vi "XYGo_example.vi"() -> ()   [LabVIEW 2016]
uses:
  Classes/Controller/Motion/A3200 Folder/A3200.lvclass
panel:
  out "Final Position":dbl[](array[numeric])
  out "Initial position":dbl[](array[numeric])
  in  "Speed (mm/s)":dbl=40.0
  in  "XY":dbl[](array[numeric])=[200.0, 300.0]
  # "Input parameter"
  # "Output Current Position"
  # "X\nY"
  # "X\nY\nZ\nU"
  # "1. This example shows how to move gantry to an absolute position on the XY plane with speed specified. \n2. The program would also show the position before and after the moving"
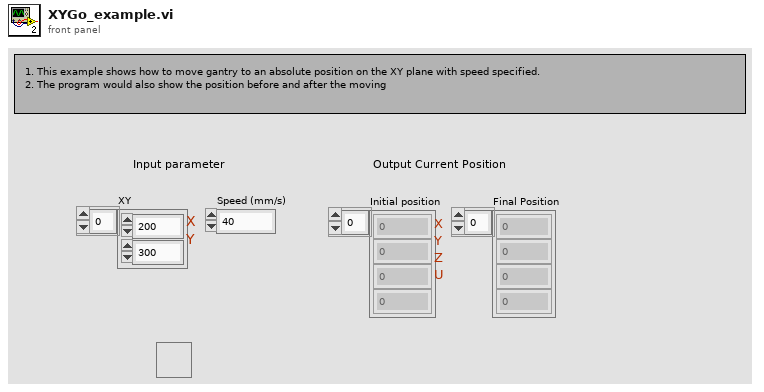
[diagram p1: front panel]
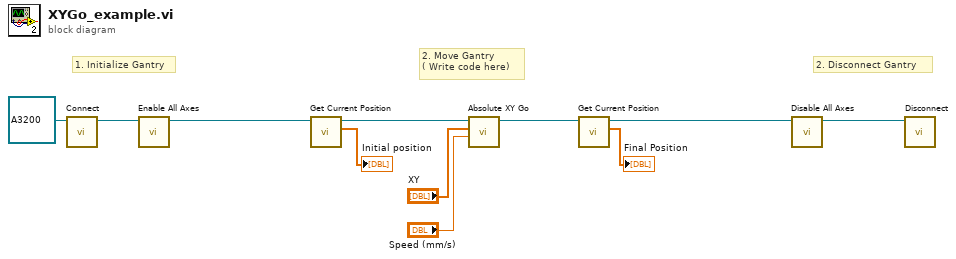
[diagram p0: block diagram]
diagram:
  # "2. Disconnect Gantry"
  # "2. Move Gantry \n( Write code here)"
  # "1. Initialize Gantry"
  n1 = call-dynamic "Connect.vi"("Gantry in"=refnum<class "A3200.lvclass"> refnum ("A3200.lvclass")) -> ("Gantry out"=w10:refnum<class "A3200.lvclass">)  [unwired: 9 in, 1 out]
  n2 = call-dynamic "Enable All Axes.vi"("A3200 in"=w10) -> ("A3200 out"=w6:refnum<class "A3200.lvclass">)  [unwired: 9 in, 1 out]
  n3 = call-dynamic "Get Current Position.vi"("Gantry in"=w6) -> ("XYZTheta Out"=→"Initial position":dbl[], "Gantry out"=w5:refnum<class "A3200.lvclass">)  [unwired: 8 in, 1 out]
  n4 = call-dynamic "Absolute XY Go.vi"("Speed"="Speed (mm/s)", "XY"="XY", "Gantry in"=w5) -> ("Gantry out"=w3:refnum<class "A3200.lvclass">)  [unwired: 7 in, 1 out]
  n5 = call-dynamic "Get Current Position.vi"("Gantry in"=w3) -> ("XYZTheta Out"=→"Final Position":dbl[], "Gantry out"=w2:refnum<class "A3200.lvclass">)  [unwired: 8 in, 1 out]
  n6 = call-dynamic "Disable All Axes.vi"("Gantry in"=w2) -> ("Gantry out"=w9:refnum<class "A3200.lvclass">)  [unwired: 9 in, 1 out]
  n7 = call-dynamic "Disconnect.vi"("Gantry in"=w9) -> ()  [unwired: 9 in, 1 out]
